vi "TelemetryDebug.vi"() -> ()   [LabVIEW 2020, in "VectoTools.lvlib" / "TelemetryDebug.lvclass"]
uses:
  TelemetryDebug/TelemetryDebug.lvclass
  TelemetryDebug/TelemetryDebug.lvclass/TelemetryDebug.ctl
panel:
  in  "Bind Address":string
  in  "Start":bool
  in  "DiscoveryPort":u16
  in  "Discovery Address":string
  in  "Cluster":string
  in  "System":string
  in  "Tree":string(tree)
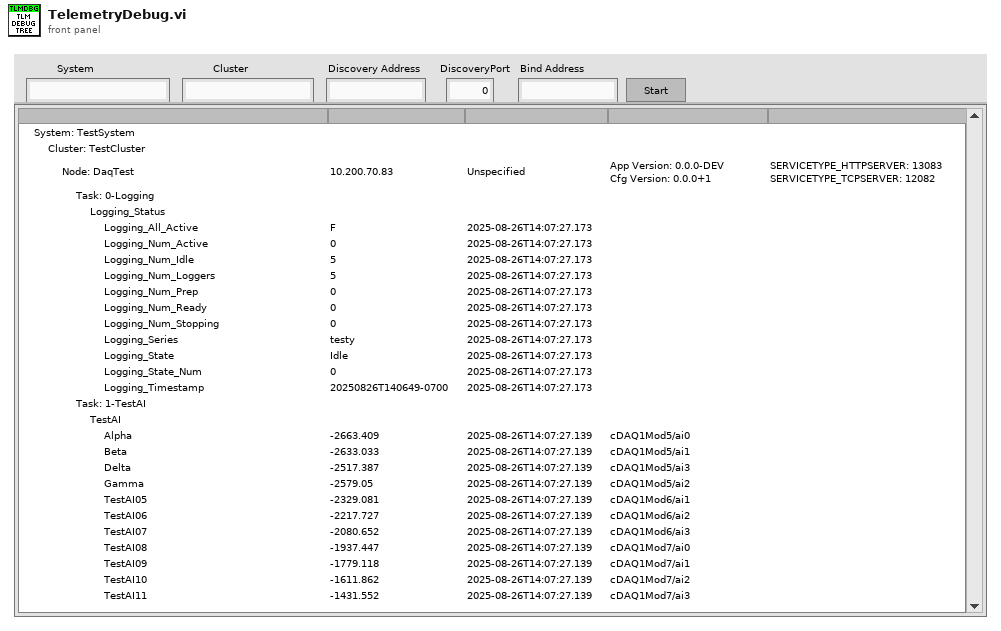
[diagram p1: front panel]
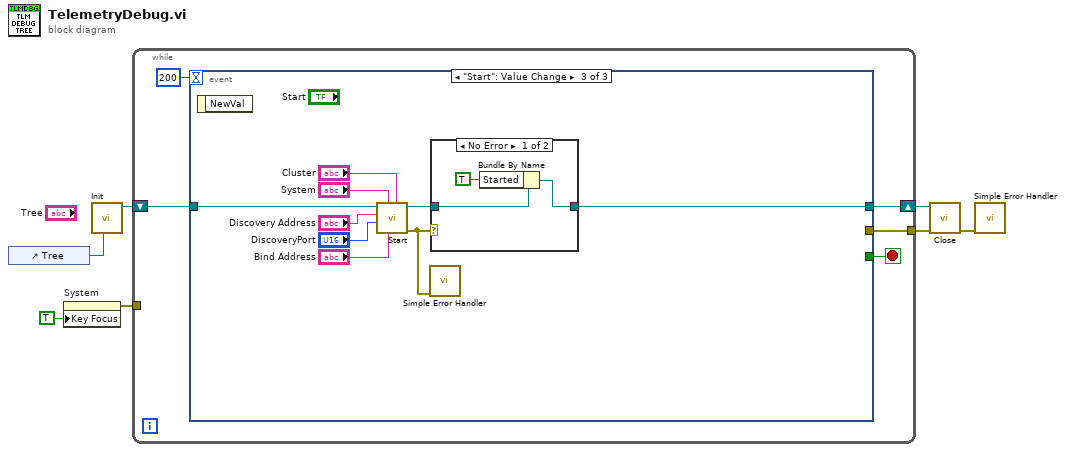
[diagram p0: block diagram]
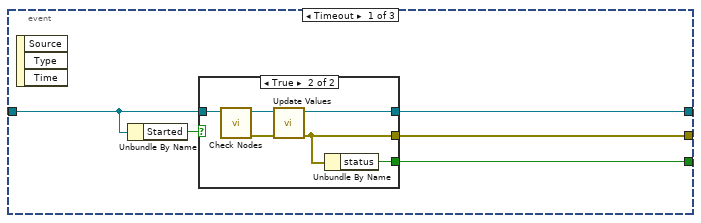
[diagram p2: hidden frame]
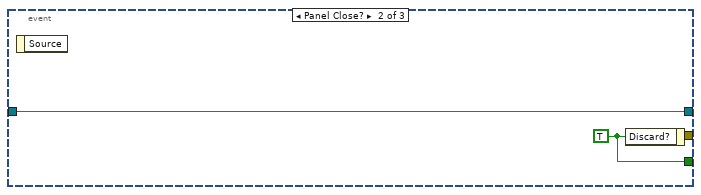
[diagram p4: hidden frame]
diagram:
  n1 = control-ref of="Tree"() -> (w4:refnum<vi>)
  n2 = property on="System" class="Str"("Key Focus"=TRUE) -> (error out=w2:errorcluster)  [unwired: 2 in, 1 out]
  n3 = call "Init.vi"("Tree"=w4) -> ("TelemetryDebug out"=w7:refnum<class "TelemetryDebug.lvclass">)  [unwired: 9 in, 1 out]
  n4 = while {
    shift-right: [w10] -> w6
    shift-left: w7 -> [w11]
    tunnel: w2 -> [_]
    tunnel: [w8] -> w1
    stop <- w9 stop-if-true
    n5 = event shown="[2] \"Start\": Value Change" {
      selector: _ -> [_ _ _]
      dyn-events: _ -> [_ _ _]
      timeout: 200 -> [_ _ _]
      tunnel: w11 -> [w14 w26 w35]
      tunnel: [w17 w26 w28] -> w10
      tunnel: [w16 w25 _] -> w9
      tunnel: [w15 _ _] -> w8
      event Timeout {
        n6 = event-data() -> ()  [unwired: 1 in, 3 out]
        n7 = Unbundle By Name(w14) -> ("Started"=w13:bool)
        n8 = case shown="True" w13 {
          tunnel: [w18 w24] -> w17
          tunnel: [_ w21] -> w16
          tunnel: [_ w20] -> w15
          tunnel: w14 -> [w18 w19]
          frame False {
          }
          frame True {
            n9 = call "Check Nodes.vi"("TelemetryDebug in"=w19) -> ("error out"=w22:errorcluster, "TelemetryDebug out"=w23:refnum<class "TelemetryDebug.lvclass">)  [unwired: 9 in]
            n10 = call "Update Values.vi"("error in (no error)"=w22, "TelemetryDebug in"=w23) -> ("error out"=w20:errorcluster, "TelemetryDebug out"=w24:refnum<class "TelemetryDebug.lvclass">)  [unwired: 8 in]
            n11 = Unbundle By Name(w20) -> ("status"=w21:bool)
          }
        }
      }
      event Panel Close? {
        w25 = TRUE ("Discard?")
        n12 = event-data() -> ()  [unwired: 1 in, 1 out]
        n13 = event-data("Discard?"=w25) -> ()  [unwired: 1 in, 1 out]
      }
      event "Start": Value Change {
        n14 = event-data() -> ()  [unwired: 1 in, 1 out]
        n15 = call "Start.vi"("Cluster"="Cluster", "Bind Address"="Bind Address", "System"="System", "DiscoveryPort"="DiscoveryPort", "Discovery Address"="Discovery Address", "TelemetryDebug in"=w35) -> ("error out"=w27:errorcluster, "TelemetryDebug out"=w34:refnum<class "TelemetryDebug.lvclass">)  [unwired: 4 in]
        n16 = call <vilib>:"Simple Error Handler.vi"("error in (no error)"=w27) -> ()  [unwired: 4 in, 5 out]
        n17 = case shown="No Error" w27 {
          tunnel: w34 -> [w38 w39]
          tunnel: [w37 w39] -> w28
          frame No Error {
            n18 = Bundle By Name(cluster=w38, "Started"=TRUE) -> (w37:refnum<class "TelemetryDebug.lvclass">)
          }
          frame Error {
          }
        }
      }
    }
  }
  n19 = call "Close.vi"("error in (no error)"=w1, "TelemetryDebug in"=w6) -> ("error out"=w5:errorcluster)  [unwired: 9 in]
  n20 = call <vilib>:"Simple Error Handler.vi"("error in (no error)"=w5) -> ()  [unwired: 4 in, 5 out]
